vi "ConfigureChannels.vi"(4 "Initial value":bool, 5 "Direction":T2, 6 "Pull up/down":T1, 7 "Channels":i32[](array[numeric]), 8 "error in":errorcluster) -> (0 "error out":errorcluster)   [LabVIEW 2014]
uses:
  controls/IO_Direction.ctl
  controls/PullUpDown.ctl
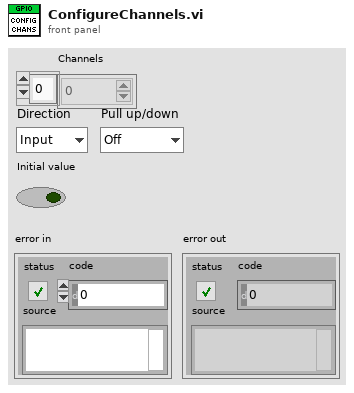
[diagram p1: front panel]
types:
  T1 = typedef "PullUpDown.ctl" = enum16{"Off", "Pull up", "Pull down"}
  T2 = typedef "IO_Direction.ctl" = enum16{"Input", "Output"}
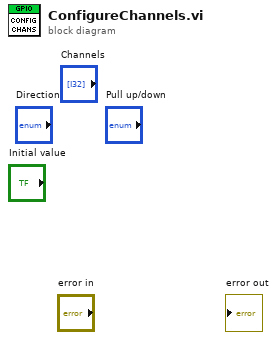
[diagram p0: block diagram]
diagram:
